vi "fpgaVI.vi"() -> ()   [LabVIEW 2020]
uses:
  <vilib>/eio/EIONode/EIONode.xnode
  <vilib>/rvi/eio/common/nirviEmuTemplateMethod_errors.vi
panel:
  in  "Mod2/AO3":fxp<+/-,20,5>
  in  "Mod2/AO2":fxp<+/-,20,5>
  in  "Mod2/AO1":fxp<+/-,20,5>
  in  "Mod2/AO0":fxp<+/-,20,5>
  in  "Mod4/AO3":fxp<+/-,20,5>
  in  "Mod4/AO2":fxp<+/-,20,5>
  in  "Mod4/AO1":fxp<+/-,20,5>
  in  "stop":bool
  out "Mod1/AI0":fxp<+/-,26,5>
  in  "Mod4/AO0":fxp<+/-,20,5>
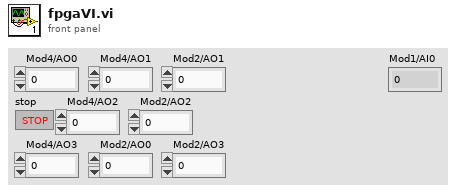
[diagram p1: front panel]
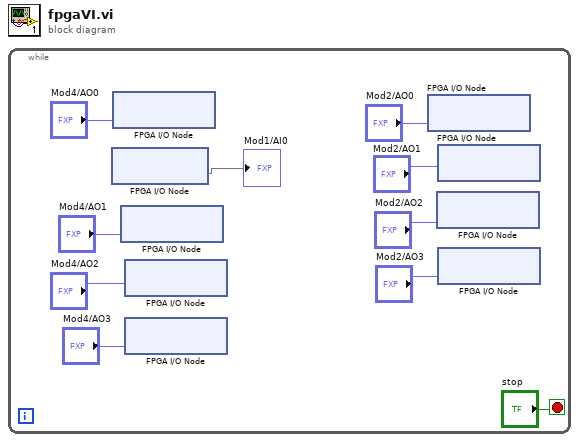
[diagram p0: block diagram]
diagram:
  n1 = while {
    stop <- "stop" stop-if-true
    n2 = xnode "FPGA I/O Node"() -> ("Mod1/AI0"=→"Mod1/AI0")  [unwired: 1 in, 1 out]
    n3 = xnode "FPGA I/O Node"("Mod4/AO0"="Mod4/AO0") -> ()  [unwired: 1 in, 1 out]
    n4 = xnode "FPGA I/O Node"("Mod4/AO1"="Mod4/AO1") -> ()  [unwired: 1 in, 1 out]
    n5 = xnode "FPGA I/O Node"("Mod4/AO2"="Mod4/AO2") -> ()  [unwired: 1 in, 1 out]
    n6 = xnode "FPGA I/O Node"("Mod4/AO3"="Mod4/AO3") -> ()  [unwired: 1 in, 1 out]
    n7 = xnode "FPGA I/O Node"("Mod2/AO0"="Mod2/AO0") -> ()  [unwired: 1 in, 1 out]
    n8 = xnode "FPGA I/O Node"("Mod2/AO2"="Mod2/AO2") -> ()  [unwired: 1 in, 1 out]
    n9 = xnode "FPGA I/O Node"("Mod2/AO1"="Mod2/AO1") -> ()  [unwired: 1 in, 1 out]
    n10 = xnode "FPGA I/O Node"("Mod2/AO3"="Mod2/AO3") -> ()  [unwired: 1 in, 1 out]
  }
